vi "Return Island Status.vi"(6 "error":string, 8 "error in (no error)":errorcluster, 9 "Status":T1, 11 "SCADA in":refnum<class "SCADA.lvclass">) -> (0 "error out":errorcluster, 3 "SCADA out":refnum<class "SCADA.lvclass">)   [LabVIEW 2015, in "SCADA Core.lvlib" / "SCADA.lvclass"]
uses:
  SCADA.lvclass
  SCADA Abstract Messages/Simple Command Status Msg/Simple Command Status.ctl
  <vilib>/ActorFramework/Actor/Actor.lvclass/Actor.ctl
  SCADA.lvclass/SCADA.ctl
  Controls/Grid Mode.ctl
  <vilib>/ActorFramework/Actor/Actor.lvclass
  SCADA Abstract Messages/Simple Command Status Msg/Simple Command Status Msg.lvclass
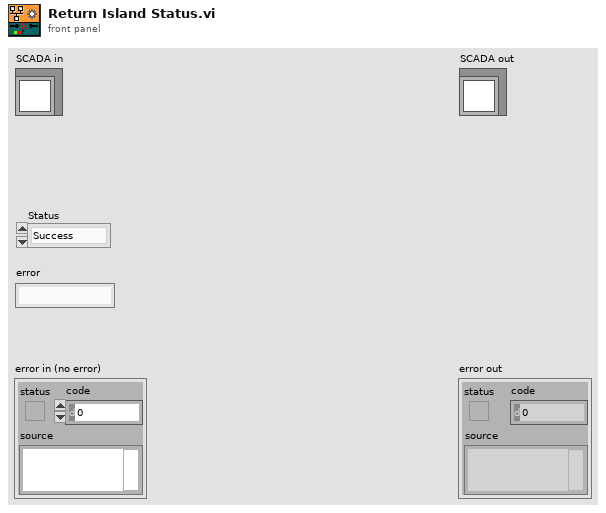
[diagram p1: front panel]
types:
  T1 = typedef "SCADA Core.lvlib/Simple Command Status Msg.lvclass/Simple Command Status.ctl" = enum16{"Success", "Failure"}
  T2 = typedef "SCADA Core.lvlib/SCADA.lvclass/Grid Mode.ctl" = enum16{"Off", "Grid Connected", "Islanded", "Synchronizing"}
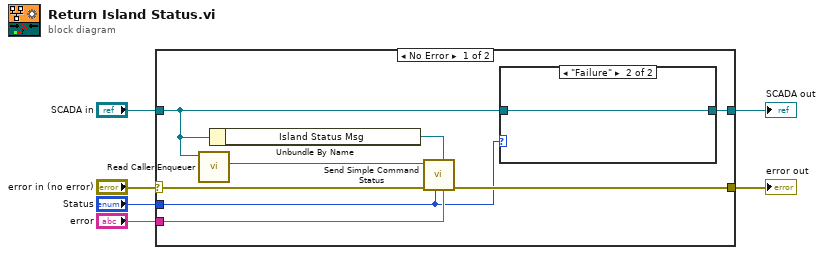
[diagram p0: block diagram]
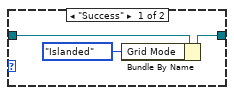
[diagram p2: hidden frame]
diagram:
  n1 = case shown="No Error" "error in (no error)" {
    selector: "error in (no error)" -> [w14 w20]
    tunnel: [w13 w20] -> w2
    tunnel: [w8 w19] -> w1
    tunnel: "SCADA in" -> [w12 w19]
    tunnel: "error" -> [w9 _]
    tunnel: "Status" -> [w7 _]
    frame No Error {
      n2 = call <vilib>:"Read Caller Enqueuer.vi"("Actor"=w12) -> ("Caller Enqueuer"=w10:refnum<class "Message Enqueuer.lvclass">)  [unwired: 10 in]
      n3 = Unbundle By Name(w12) -> ("Island Status Msg"=w11:refnum<class "Simple Command Status Msg.lvclass">)
      n4 = call "Send Simple Command Status.vi"("error"=w9, "Simple Command Status Msg"=w11, "Status"=w7, "error in (no error)"=w14, "Message Enqueuer in"=w10) -> ("error out"=w13:errorcluster)  [unwired: 5 in, 1 out]
      n5 = case shown="\"Failure\"" w7 {
        tunnel: w12 -> [w17 w18]
        tunnel: [w16 w18] -> w8
        frame "Success" {
          n6 = Bundle By Name(cluster=w17, "Grid Mode"=Grid_Mode."Islanded") -> (w16:refnum<class "SCADA.lvclass">)
        }
        frame "Failure" {
        }
      }
    }
    frame Error {
    }
  }
  "error out" <- w2
  "SCADA out" <- w1
